vi "Set Source Property.vi"(5 "Property Index":i32, 7 "Source Index":i32, 8 "error in (no error)":errorcluster, 9 "Property Value":variant, 10 "Property Name":string, 11 "BuildSpec in":refnum<vi>) -> (0 "error out":errorcluster, 3 "BuildSpec out":refnum<vi>)   [LabVIEW 2019, in "Project Sync Tools.lvclass"]
uses:
  Project Sync Tools.lvclass
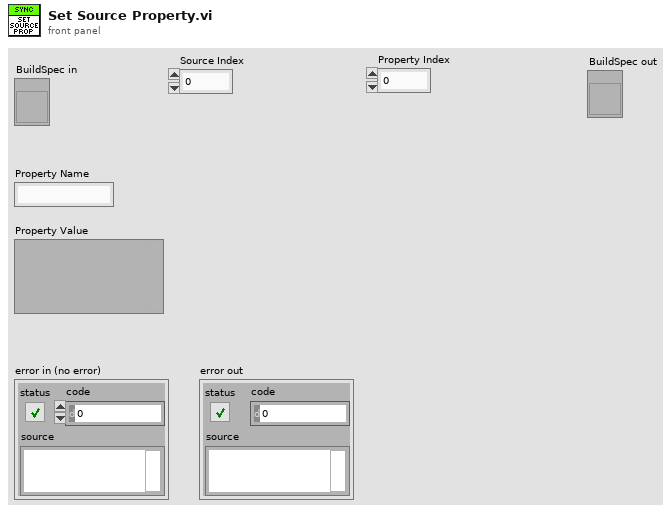
[diagram p1: front panel]
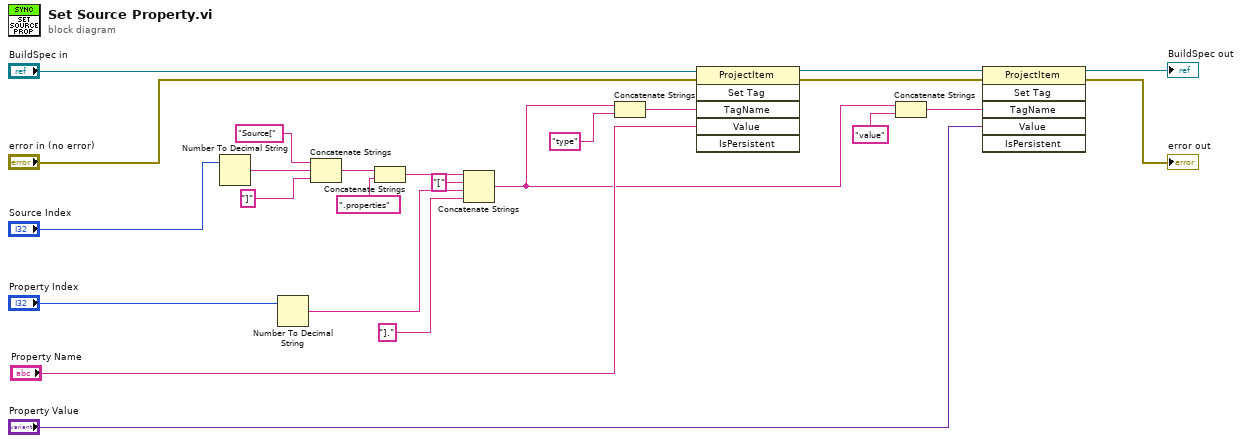
[diagram p0: block diagram]
diagram:
  n1 = Number To Decimal String(number="Source Index") -> (decimal integer string=w5:string)  [unwired: 1 in]
  n2 = Number To Decimal String(number="Property Index") -> (decimal integer string=w15:string)  [unwired: 1 in]
  n3 = Concatenate Strings("Source[" ("string"), w5, "]") -> (w3:string)
  n4 = Concatenate Strings(w3, ".properties") -> (w14:string)
  n5 = Concatenate Strings(w14, "[" ("string"), w15, "]." ("string")) -> (w2:string)
  n6 = Concatenate Strings(w2, "type" ("string")) -> (w11:string)
  n7 = invoke class="ProjectItem" method="Set Tag"(reference="BuildSpec in", error in="error in (no error)", "TagName"=w11, "Value"="Property Name") -> (reference out=w18:refnum<vi>, error out=w19:errorcluster)  [unwired: 2 in, 4 out]
  n8 = Concatenate Strings(w2, "value" ("string")) -> (w21:string)
  n9 = invoke class="ProjectItem" method="Set Tag"(reference=w18, error in=w19, "TagName"=w21, "Value"="Property Value") -> (reference out=→"BuildSpec out":refnum<vi>, error out=→"error out":errorcluster)  [unwired: 2 in, 4 out]
